vi "flight_time.vi"() -> ()   [LabVIEW 2013]
uses:
  <vilib>/Instr/_visa.llb/VISA Configure Serial Port (Instr).vi
  <vilib>/Analysis/NI_AALBase.lvlib
panel:
  in  "?":bool
  out "time":dbl
  in  "high_time":i32
  in  "low_time":i32
  out "diferença":dbl
  out "high_time":dbl format="%#_10g"
  out "low_time":dbl format="%#_10g"
  in  "stop":bool
  in  "high":u32
  in  "low":i32
  in  "Pcell1":u32[](array[numeric])
  in  "Pcell2":u32[](array[numeric])
  in  "Pcell3":u32[](array[numeric])
  in  "Pcell4":u32[](array[numeric])
  in  "last":u32
  out "time":u32[](graph)
  in  "Tab Control":enum32{"raw data", "filter", "weight"}(tab)
  out "celula 4":i32(graph)
  out "celula 3":i32(graph)
  out "celula 2":i32(graph)
  out "celula 1":i32(graph)
  out "peso_cell2":dbl[](graph) caption="Sine"
  out "peso_cell3":dbl[](graph) caption="Sine"
  out "peso_cell4":dbl[](graph) caption="Sine"
  out "peso_cell1":dbl[](graph) caption="Sine"
  out "cell":u8[](array[numeric])
  out "output_int16":i32[](array[numeric])
  out "data":u8[](array[numeric])
  in  "serial_port":refnum<visa-resource-name> caption="Porta Serial"
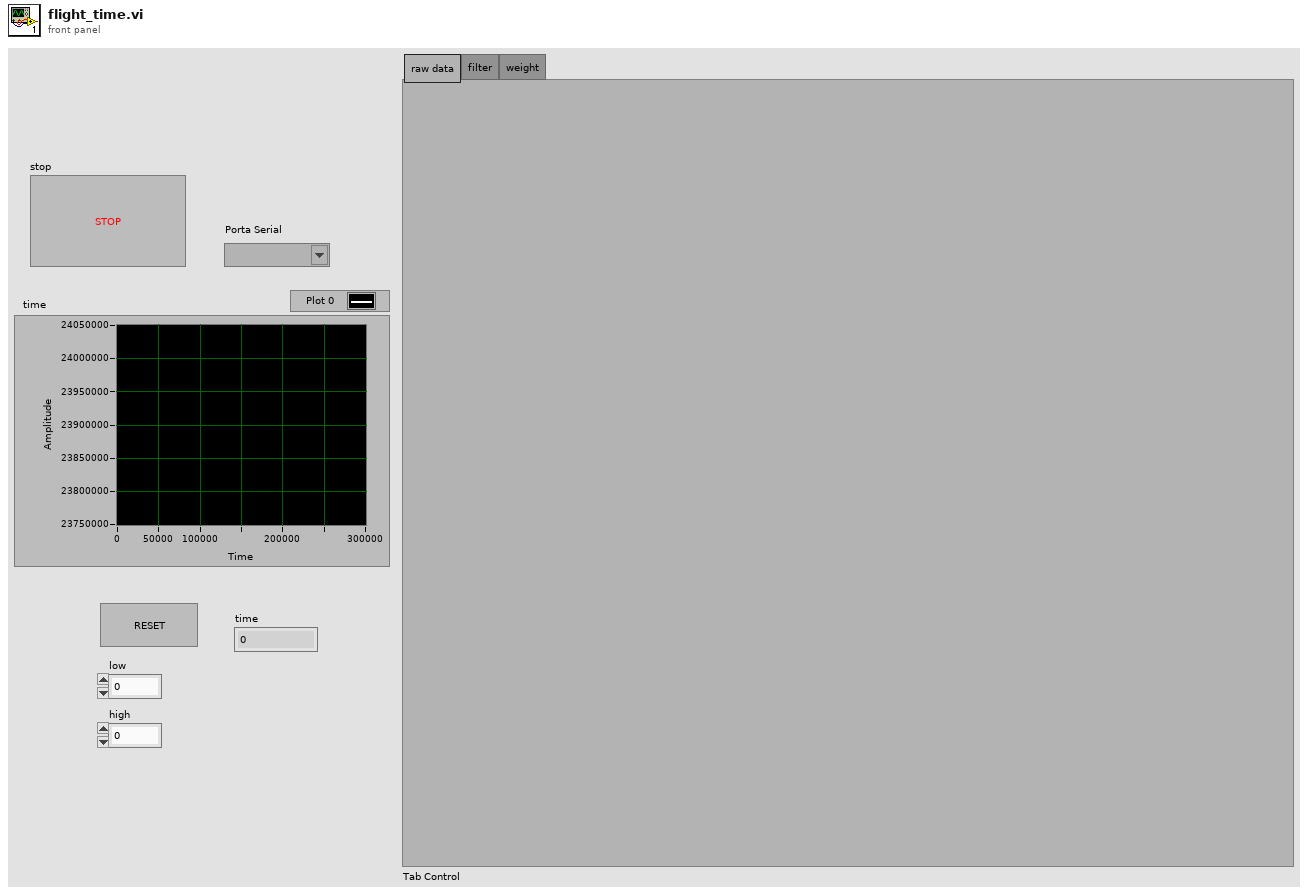
[diagram p1: front panel]
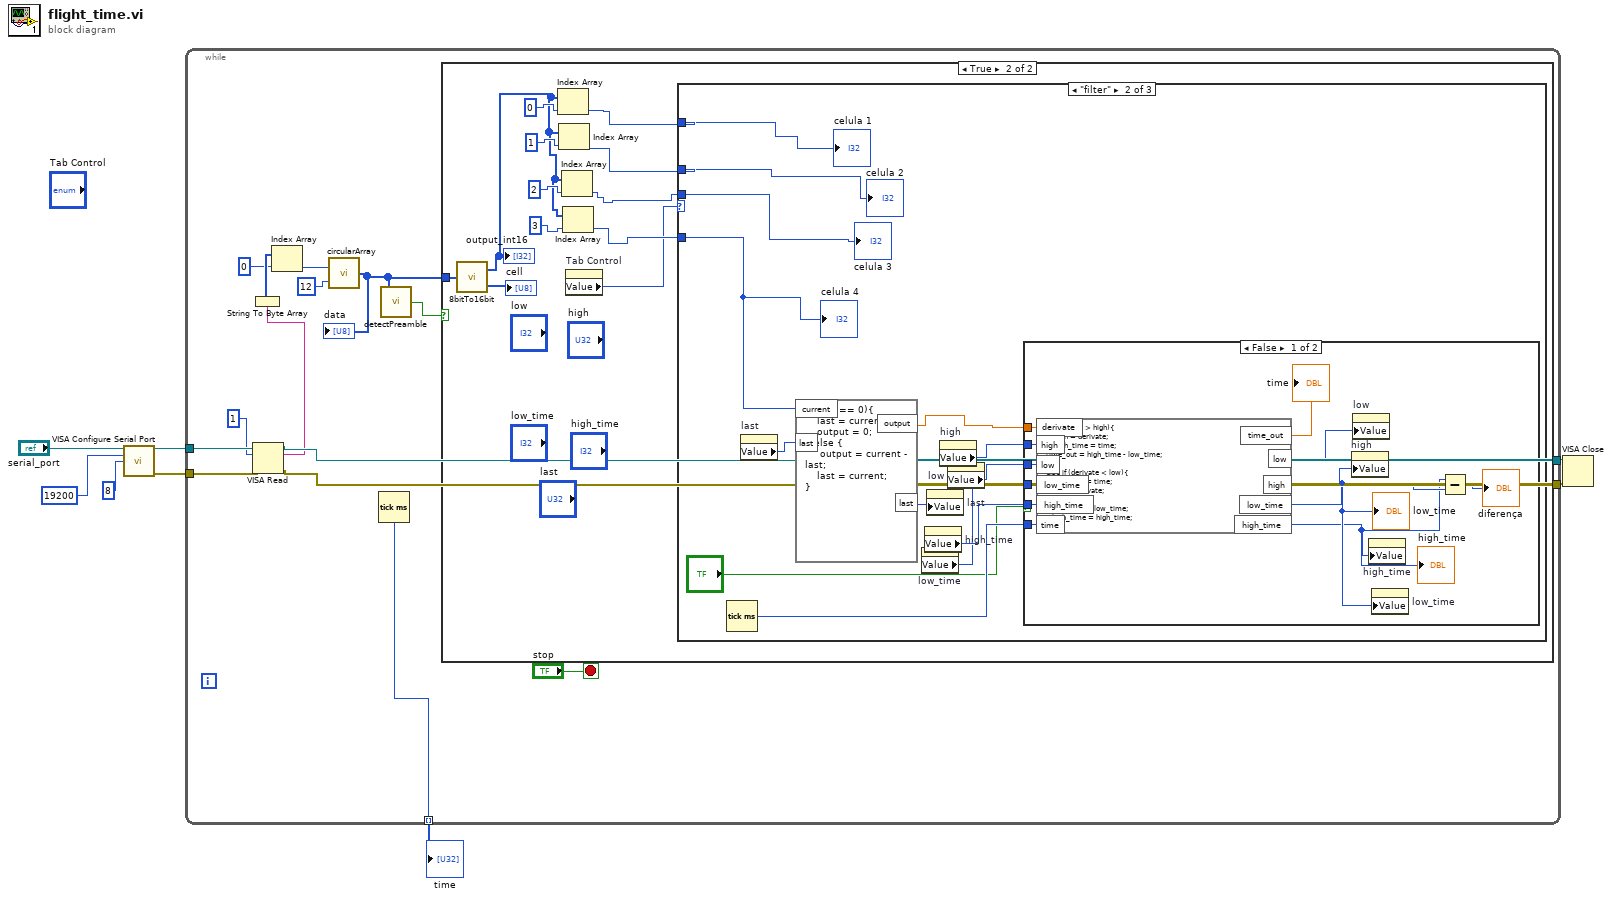
[diagram p0: block diagram]
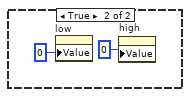
[diagram p4: hidden frame]
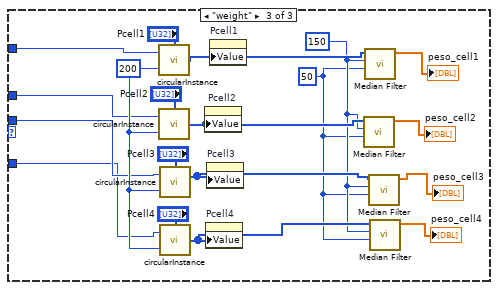
[diagram p5: hidden frame]
diagram:
  n1 = call-poly "VISA Configure Serial Port"("VISA resource name"="serial_port", "baud rate (9600)"=u32 19200, "data bits (8)"=u16 8) -> ("VISA resource name out"=w5:refnum<visa-resource-name>, "error out"=w4:errorcluster)  [unwired: 11 in]
  n2 = while {
    tunnel: w5 -> [w22]
    tunnel: w4 -> [w21]
    tunnel: [w19] -> w2
    tunnel: [w20] -> w3
    tunnel: [w10] -> w1 mode=indexing
    stop <- "stop" stop-if-true
    n3 = VISA Read(VISA resource name=w22, byte count=1, error in (no error)=w21) -> (VISA resource name out=w20:refnum<visa-resource-name>, read buffer=w14:string, error out=w19:errorcluster)  [unwired: 1 out]
    n4 = String To Byte Array(string=w14) -> (unsigned byte array=w17:u8[])
    n5 = Index Array(array=w17, index=0) -> (element=w11:u8)
    n6 = call "circularArray.vi"("max-size"=u8 12, "element"=w11) -> ("dataout"=w12:u8[])
    "data" <- w12
    n7 = Tick Count (ms)() -> (millisecond timer value=w10:u32)
    n8 = call "detectPreamble.vi"("data-in"=w12) -> ("detected"=w9:bool)
    n9 = case shown="True" w9 {
      tunnel: w12 -> [_ w33]
      frame False {
      }
      frame True {
        n10 = call "8bitTo16bit.vi"("input_byte"=w33) -> ("output_int16"=w28:i32[], "cell"=→"cell":u8[])
        "output_int16" <- w28
        n11 = Index Array(array=w28, index=0) -> (element=w24:i32)
        n12 = Index Array(array=w28, index=1) -> (element=w25:i32)
        n13 = Index Array(array=w28, index=2) -> (element=w26:i32)
        n14 = Index Array(array=w28, index=3) -> (element=w27:i32)
        n15 = property on="Tab Control" class="TabCtl (strict)"() -> ("Value"=w23:enum32{"raw data", "filter", "weight"})  [unwired: 2 in, 2 out]
        n16 = case shown="\"filter\"" w23 {
          tunnel: w24 -> [_ w38 w75]
          tunnel: w25 -> [_ w36 w74]
          tunnel: w26 -> [_ w37 w73]
          tunnel: w27 -> [_ w35 w72]
          frame "raw data", Default {
          }
          frame "filter" {
            n17 = Tick Count (ms)() -> (millisecond timer value=w40:u32)
            n18 = property on="last" class="DigNum (strict)"() -> ("Value"=w47:u32)  [unwired: 2 in, 2 out]
            n19 = formula code="if (last == 0){\n    last = current;\n    output = 0;\n} else {\n     output = current - last;\n    last = current;\n}"("last"=w47, "current"=w35) -> ("output"=w45:dbl, "last"=w46:u32)
            n20 = property on="low_time" class="DigNum (strict)"() -> ("Value"=w41:i32)  [unwired: 2 in, 2 out]
            n21 = property on="high_time" class="DigNum (strict)"() -> ("Value"=w42:i32)  [unwired: 2 in, 2 out]
            n22 = property on="last" class="DigNum (strict)"("Value"=w46) -> ()  [unwired: 2 in, 2 out]
            n23 = property on="high" class="DigNum (strict)"() -> ("Value"=w44:u32)  [unwired: 2 in, 2 out]
            n24 = property on="low" class="DigNum (strict)"() -> ("Value"=w43:i32)  [unwired: 2 in, 2 out]
            n25 = case shown="False" "?" {
              tunnel: w45 -> [w59 _]
              tunnel: w44 -> [w58 _]
              tunnel: w43 -> [w57 _]
              tunnel: w42 -> [w53 _]
              tunnel: w41 -> [w52 _]
              tunnel: w40 -> [w49 _]
              frame False {
                n26 = formula code="if (derivate > high){\n    high = derivate;\n    high_time = time;\ntime_out = high_time - low_time;\n}\nelse if (derivate < low){\n   low_time = time;\n   low = derivate;  \n} else {\n   low_time = low_time;\n   high_time = high_time;\n}"("derivate"=w59, "high"=w58, "low"=w57, "time"=w49, "low_time"=w52, "high_time"=w53) -> ("low"=w56:i32, "high"=w55:u32, "low_time"=w51:i32, "high_time"=w50:i32, "time_out"=→"time":dbl)
                "low_time" <- w51
                "high_time" <- w50
                n27 = property on="high" class="DigNum (strict)"("Value"=w55) -> ()  [unwired: 2 in, 2 out]
                n28 = property on="low" class="DigNum (strict)"("Value"=w56) -> ()  [unwired: 2 in, 2 out]
                n29 = property on="high_time" class="DigNum (strict)"("Value"=w50) -> ()  [unwired: 2 in, 2 out]
                n30 = property on="low_time" class="DigNum (strict)"("Value"=w51) -> ()  [unwired: 2 in, 2 out]
                n31 = Subtract(x=w50, y=w51) -> (x-y=→"diferença":i32)
              }
              frame True {
                n32 = property on="low" class="DigNum (strict)"("Value"=0 ("low")) -> ()  [unwired: 2 in, 2 out]
                n33 = property on="high" class="DigNum (strict)"("Value"=u32 0 ("high")) -> ()  [unwired: 2 in, 2 out]
              }
            }
            "celula 1" <- w38
            "celula 2" <- w36
            "celula 3" <- w37
            "celula 4" <- w35
          }
          frame "weight" {
            w66 = 50 ("left rank")
            w67 = 150 ("left rank")
            w78 = i16 200 ("max-size")
            n34 = call "circularInstance.vi"("data"="Pcell1", "max-size"=w78, "element"=w75) -> ("dataout"=w71:u32[])
            n35 = call "circularInstance.vi"("data"="Pcell2", "max-size"=w78, "element"=w74) -> ("dataout"=w70:u32[])
            n36 = call "circularInstance.vi"("data"="Pcell3", "max-size"=w78, "element"=w73) -> ("dataout"=w69:u32[])
            n37 = call "circularInstance.vi"("data"="Pcell4", "max-size"=w78, "element"=w72) -> ("dataout"=w68:u32[])
            n38 = property on="Pcell2" class="Arr (strict)"("Value"=w70) -> ()  [unwired: 2 in, 2 out]
            n39 = property on="Pcell4" class="Arr (strict)"("Value"=w68) -> ()  [unwired: 2 in, 2 out]
            n40 = property on="Pcell3" class="Arr (strict)"("Value"=w69) -> ()  [unwired: 2 in, 2 out]
            n41 = property on="Pcell1" class="Arr (strict)"("Value"=w71) -> ()  [unwired: 2 in, 2 out]
            n42 = call <vilib>:"Median Filter.vi"("right rank"=w66, "left rank"=w67, "X"=w70) -> ("Filtered X"=→"peso_cell2":dbl[])  [unwired: 7 in, 1 out]
            n43 = call <vilib>:"Median Filter.vi"("right rank"=w66, "left rank"=w67, "X"=w71) -> ("Filtered X"=→"peso_cell1":dbl[])  [unwired: 7 in, 1 out]
            n44 = call <vilib>:"Median Filter.vi"("right rank"=w66, "left rank"=w67, "X"=w69) -> ("Filtered X"=→"peso_cell3":dbl[])  [unwired: 7 in, 1 out]
            n45 = call <vilib>:"Median Filter.vi"("right rank"=w66, "left rank"=w67, "X"=w68) -> ("Filtered X"=→"peso_cell4":dbl[])  [unwired: 7 in, 1 out]
          }
        }
      }
    }
  }
  "time" <- w1
  n46 = VISA Close(VISA resource name=w3, error in (no error)=w2) -> ()  [unwired: 1 out]
